vi "Open DSF Configuration Data.vi"(8 "error in (no error)":errorcluster, 9 "replace if found? (F)":bool, 10 "create file if necessary (T)":bool=TRUE, 11 "dsf configuration file path":path) -> (0 "error out":errorcluster, 1 "file replaced?":bool, 2 "file created?":bool, 3 "Configuration Session":refnum<class "Configuration Session.lvclass">, 4 "version":T1)   [LabVIEW 2017, in "DSF Core.lvlib" / "Configuration Session.lvclass"]
doc: "Opens a reference to the configuration data found in a platform-independent configuration file."
uses:
  Configuration Session.lvclass
  Controls/DSF Version Info.ctl
  Private/Controls/Session/DSF Config Data.ctl
  Private/Controls/DSF File Format/Internal DSF Configuration.ctl
  Private/Controls/DSF File Format/Internal DSF Plugin with ID.ctl
  Private/Controls/DSF File Format/Internal DSF Plugin Info.ctl
  Controls/DSF Timing Info.ctl
  Private/Controls/DSF File Format/Internal DSF Group with ID.ctl
  Private/Controls/DSF File Format/Internal DSF Group Info.ctl
  Private/Controls/DSF File Format/Internal DSF Transfer with ID.ctl
  Private/Controls/DSF File Format/Internal DSF Transfer Info.ctl
  Private/Controls/DSF File Format/Internal DSF Channel with ID.ctl
  Private/Controls/DSF File Format/Internal DSF Channel Info.ctl
  Private/Controls/DSF File Format/Internal DSF Settings with ID.ctl
  Private/Controls/DSF File Format/Internal DSF Settings Info.ctl
  Configuration Session.lvclass/Configuration Session.ctl
  DSF Core.lvlib
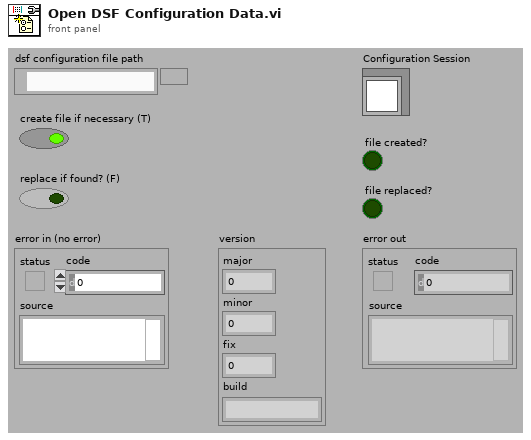
[diagram p1: front panel]
types:
  T1 = typedef "DSF Core.lvlib/DSF Version Info.ctl" = cluster{"major":u32, "minor":u32, "fix":u32, "build":string}
  T2 = typedef "DSF Core.lvlib/Configuration Session.lvclass/DSF Config Data.ctl" = cluster{"dsf configuration":T3, "path":path, "dirty":bool}
  T3 = typedef "DSF Core.lvlib/Configuration Session.lvclass/Internal DSF Configuration.ctl" = cluster{"dsfversion":T1, "version":T1, "plugins":T4[], "groups":T7[], "transfers":T9[], "channels":T11[], "settings":T13[]}
  T4 = typedef "DSF Core.lvlib/Configuration Session.lvclass/Internal DSF Plugin with ID.ctl" = cluster{"id":string, "values":T5}
  T5 = typedef "DSF Core.lvlib/Configuration Session.lvclass/Internal DSF Plugin Info.ctl" = cluster{"type":string, "timing":T6, "group ids":string[], "settings id":string, "thread count":i32}
  T6 = typedef "DSF Core.lvlib/DSF Timing Info.ctl" = cluster{"priority":u64, "decimation":u64, "offset":u64}
  T7 = typedef "DSF Core.lvlib/Configuration Session.lvclass/Internal DSF Group with ID.ctl" = cluster{"id":string, "values":T8}
  T8 = typedef "DSF Core.lvlib/Configuration Session.lvclass/Internal DSF Group Info.ctl" = cluster{"direction":i32, "timing":T6, "transfer ids":string[], "settings id":string}
  T9 = typedef "DSF Core.lvlib/Configuration Session.lvclass/Internal DSF Transfer with ID.ctl" = cluster{"id":string, "values":T10}
  T10 = typedef "DSF Core.lvlib/Configuration Session.lvclass/Internal DSF Transfer Info.ctl" = cluster{"byte order":i32, "channel ids":string[], "settings id":string}
  T11 = typedef "DSF Core.lvlib/Configuration Session.lvclass/Internal DSF Channel with ID.ctl" = cluster{"id":string, "values":T12}
  T12 = typedef "DSF Core.lvlib/Configuration Session.lvclass/Internal DSF Channel Info.ctl" = cluster{"count":u64, "buffer offset":u64, "data type":i32, "settings id":string}
  T13 = typedef "DSF Core.lvlib/Configuration Session.lvclass/Internal DSF Settings with ID.ctl" = cluster{"id":string, "values":T14}
  T14 = typedef "DSF Core.lvlib/Configuration Session.lvclass/Internal DSF Settings Info.ctl" = cluster{"key":string, "value":string}[]
  T15 = typedef "DSF Core.lvlib/Configuration Session.lvclass/DSF Config Data Ref.ctl" = refnum<data-value>
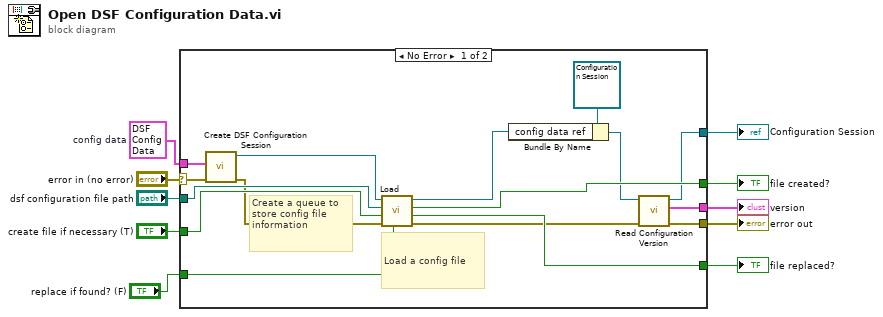
[diagram p0: block diagram]
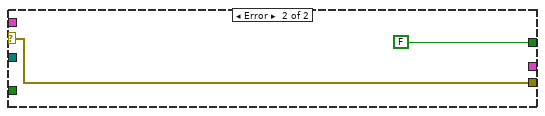
[diagram p2: hidden frame]
diagram:
  w5 = T2 {"dsf configuration"={"dsfversion"={"major"=0, "minor"=0, "fix"=0, "build"=""}, "version"={"major"=0, "minor"=0, "fix"=0, "build"=""}, "plugins"=[], "groups"=[], "transfers"=[], "channels"=[], "settings"=[]}, "path"=path "", "dirty"=FALSE}  # config data
  n1 = case shown="No Error" "error in (no error)" {
    selector: "error in (no error)" -> [w23 w28]
    tunnel: "dsf configuration file path" -> [w26 _]
    tunnel: "create file if necessary (T)" -> [w25 _]
    tunnel: [w24 FALSE ("file created?")] -> w6
    tunnel: [w11 w28] -> w7
    tunnel: w5 -> [w19 _]
    tunnel: [w14 _] -> w4
    tunnel: "replace if found? (F)" -> [w21 _]
    tunnel: [w20 _] -> w2
    tunnel: [w12 _] -> w1
    frame No Error {
      # "Load a config file"
      # "Create a queue to store config file information"
      n2 = call "Create DSF Configuration Session.vi"("error in (no error)"=w23, "config data"=w19) -> ("error out"=w22:errorcluster, "config data ref"=w18:T15)  [unwired: 8 in]
      n3 = call "Load.vi"("replace if found? (F)"=w21, "error in (no error)"=w22, "create file if necessary? (T)"=w25, "configuration file path"=w26, "config data ref in"=w18) -> ("error out"=w13:errorcluster, "file replaced?"=w20:bool, "file created?"=w24:bool, "config data ref out"=w16:T15)  [unwired: 3 out]
      n4 = Bundle By Name(cluster=refnum<class "Configuration Session.lvclass"> refnum ("Configuration Session in"), "config data ref"=w16) -> (w15:refnum<class "Configuration Session.lvclass">)
      n5 = call "Read Configuration Version.vi"("error in (no error)"=w13, "Configuration Session in"=w15) -> ("error out"=w11:errorcluster, "version"=w14:T1, "Configuration Session out"=w12:refnum<class "Configuration Session.lvclass">)  [unwired: 7 in]
    }
    frame Error {
    }
  }
  "error out" <- w7
  "file created?" <- w6
  "version" <- w4
  "file replaced?" <- w2
  "Configuration Session" <- w1
